vi "PID2 Output FGV.vi"(7 "Write":bool, 8 "error in (no error)":errorcluster, 11 "PID2 Output In (%)":dbl) -> (0 "error out":errorcluster, 3 "PID2 Output Out (%)":dbl)   [LabVIEW 2021]
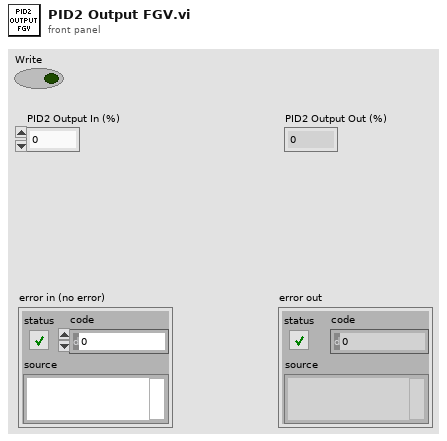
[diagram p1: front panel]
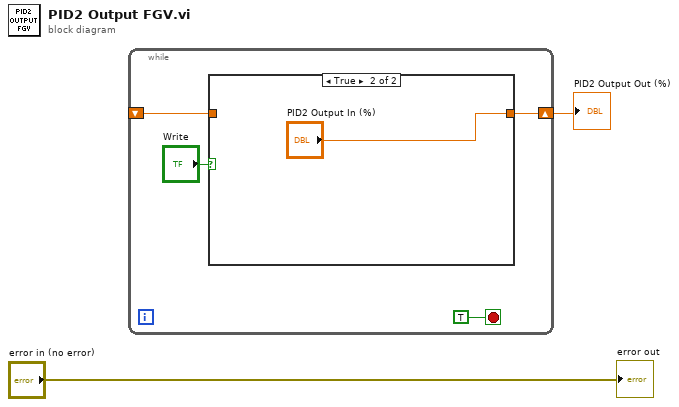
[diagram p0: block diagram]
diagram:
  n1 = while {
    shift-right: [w4] -> w2
    shift-left: _ -> [w3]
    stop <- TRUE stop-if-true
    n2 = case shown="True" "Write" {
      tunnel: [w7 "PID2 Output In (%)"] -> w4
      tunnel: w3 -> [w7 _]
      frame False {
      }
      frame True {
      }
    }
  }
  "PID2 Output Out (%)" <- w2
  "error out" <- "error in (no error)"
